vi "ziModGetNodeValueVector.vi"(0 "ModHandle In":T2 {"ModHandle" format="0x%08x"; "Conn" format="0x%08x"}, 7 "Path":string, 11 "error in":errorcluster) -> (4 "ModHandle Out":T2 {"ModHandle" format="0x%08x"; "Conn" format="0x%08x"}, 8 "VectorWave Out":T1, 15 "error out":errorcluster)   [LabVIEW 2009, in "Zurich Instruments LabOne.lvlib"]
uses:
  <instrlib>/Zurich Instruments LabOne/Zurich Instruments LabOne.lvlib
  <instrlib>/Zurich Instruments LabOne/Public/Modules/ziTypeModHandle.ctl
  <instrlib>/Zurich Instruments LabOne/Public/Data/ziTypeCoreVectorWave.ctl
  <instrlib>/Zurich Instruments LabOne/Private/ziLV32.dll
panel:
  in  "VectorWave In":T1
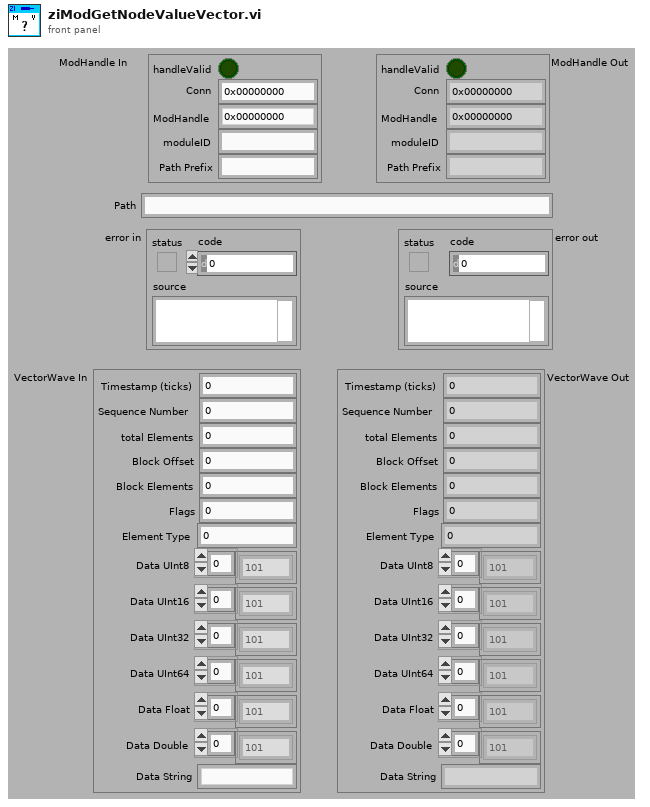
[diagram p1: front panel]
types:
  T1 = typedef "Zurich Instruments LabOne.lvlib/ziTypeCoreVectorWave.ctl" = cluster{"Timestamp (ticks)":u64, "Sequence Number":u32, "total Elements":u64, "Block Offset":u64, "Block Elements":u32, "Flags":u8, "Element Type":u8, "Data UInt8":u8[], "Data UInt16":u16[], "Data UInt32":u32[], "Data UInt64":u64[], "Data Float":sgl[], "Data Double":dbl[], "Data String":string}
  T2 = typedef "Zurich Instruments LabOne.lvlib/ziTypeModHandle.ctl" = cluster{"handleValid":bool, "Conn":u64, "ModHandle":u64, "moduleID":string, "Path Prefix":string}
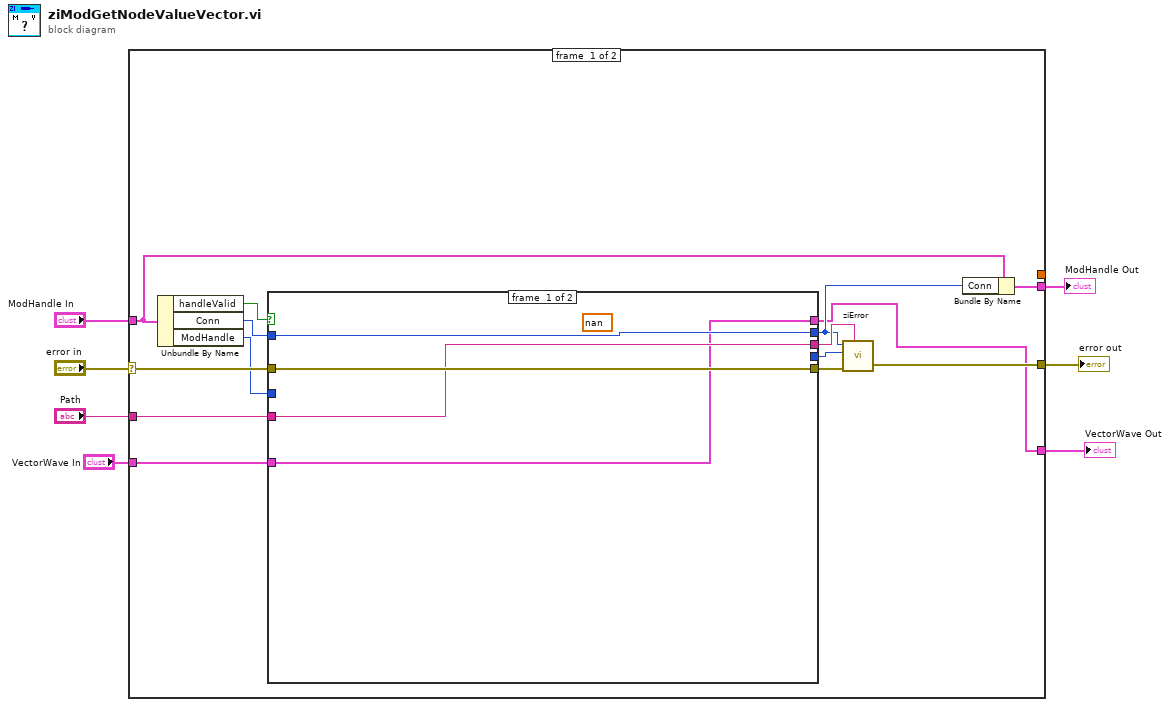
[diagram p0: block diagram]
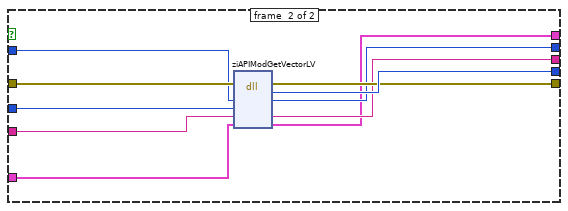
[diagram p2: hidden frame]
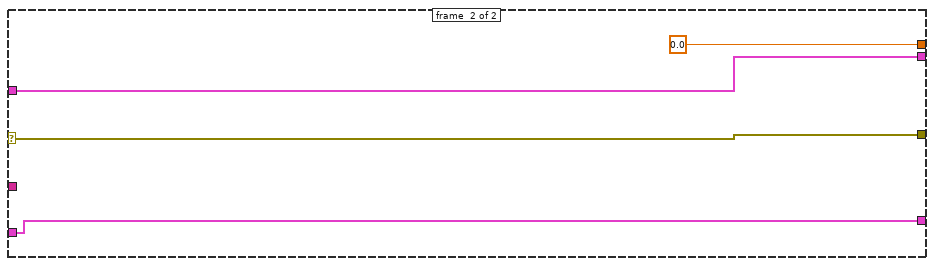
[diagram p3: hidden frame]
diagram:
  n1 = case shown="No Error" "error in" {
    selector: "error in" -> [w18 w39]
    tunnel: [w9 w39] -> w7
    tunnel: [w19 w38] -> w3
    tunnel: "ModHandle In" -> [w13 w38]
    tunnel: "Path" -> [w14 _]
    tunnel: [_ 0.0 ("Value")] -> _
    tunnel: "VectorWave In" -> [w10 w36]
    tunnel: [w8 w36] -> w1
    frame #0 {
      n2 = Unbundle By Name(w13) -> ("handleValid"=w11:bool, "Conn"=w16:u64, "ModHandle"=w12:u64)
      n3 = case shown="False" w11 {
        tunnel: [_ w35] -> w21
        tunnel: [w25 w34] -> w20
        tunnel: w18 -> [w25 w33]
        tunnel: [w23 w32] -> w17
        tunnel: w16 -> [w24 w31]
        tunnel: [w24 w30] -> w15
        tunnel: w14 -> [w23 w29]
        tunnel: w12 -> [_ w28]
        tunnel: [w22 w27] -> w8
        tunnel: w10 -> [w22 w26]
        frame #0 {
          (unwired) nan ("Value")
        }
        frame #1 {
          n4 = dll-call lib="C:/Program Files (x86)/National Instruments/LabVIEW 2009/instr.lib/Zurich Instruments LabOne/Private/ziLV*.*" fn="ziAPIModGetVectorLV"(error in=w33, "Conn"=w31, "ModHandle"=w28, "Path"=w29, w26) -> (error out=w34:errorcluster, "return type"=w35:u32, "Conn"=w30:u64, "Path"=w32:string, w27:T1)  [unwired: 3 in, 1 out]
        }
      }
      n5 = call <instrlib>:"ziError.vi"("Conn"=w15, "ziErrorCode"=w21, "Error In"=w20, "Annotation"=w17) -> ("Error Out"=w9:errorcluster)  [unwired: 2 in]
      n6 = Bundle By Name(cluster=w13, "Conn"=w15) -> (w19:T2)
    }
    frame #1 {
    }
  }
  "error out" <- w7
  "ModHandle Out" <- w3
  "VectorWave Out" <- w1
